vi "OPCServerSettings.vi"() -> (0 "OK Button 2":bool)   [LabVIEW 2025]
uses:
  <vilib>/Utility/config.llb/NI_LVConfig.lvlib
  <vilib>/Utility/config.llb/Write Key (String).vi
  <vilib>/Utility/config.llb/Read Key (String).vi
panel:
  in  "Cluster":cluster{"serverUrl":string, "nodeid":string}
  in  "Cancel Button":bool
  in  "OK Button":bool
  # "OPC Server settings"
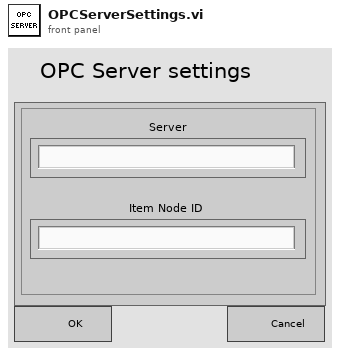
[diagram p1: front panel]
types:
  T1 = typedef "NI_LVConfig.lvlib/Config Data RefNum.ctl" = refnum<k1>
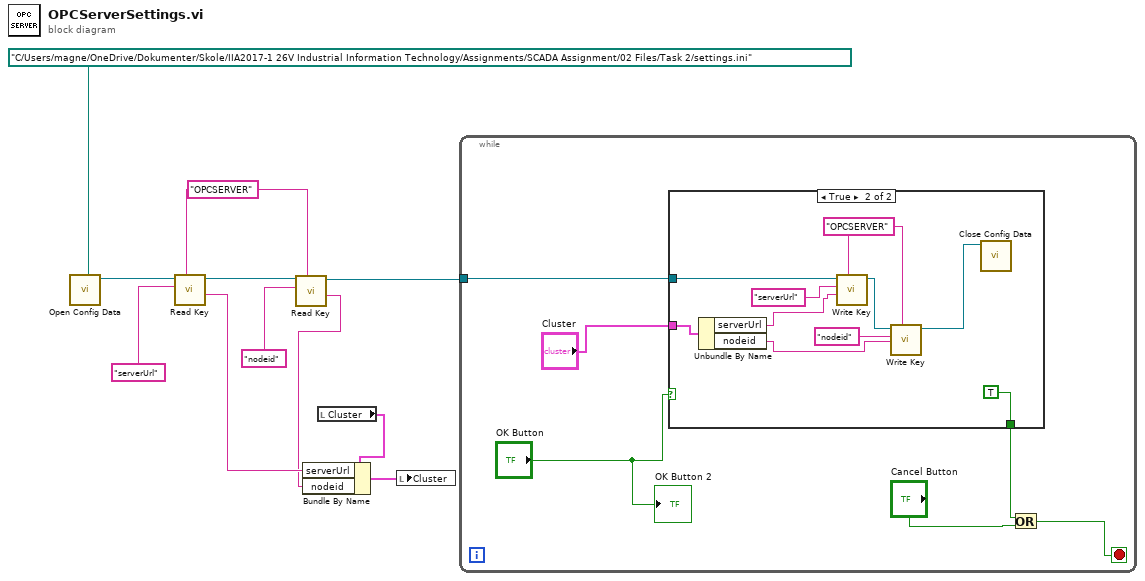
[diagram p0: block diagram]
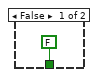
[diagram p2: hidden frame]
diagram:
  w10 = "OPCSERVER" ("section")
  n1 = call <vilib>:"Open Config Data.vi"("configuration file path"=path "C:/Users/magne/OneDrive/Dokumenter/Skole/IIA2017-1 26V Industrial Information Technology/Assignments/SCADA Assignment/02 Files/Task 2/settings.ini") -> ("refnum"=w9:T1)  [unwired: 8 in, 2 out]
  n2 = call-poly <vilib>:"Read Key.vi"("section"=w10, "key"="serverUrl", "refnum"=w9) -> ("value"=w4:string, "refnum out"=w8:T1)  [unwired: 5 in, 2 out]
  n3 = call-poly <vilib>:"Read Key.vi"("section"=w10, "key"="nodeid", "refnum"=w8) -> ("value"=w3:string, "refnum out"=w7:T1)  [unwired: 5 in, 2 out]
  n4 = local read "Cluster"() -> (w6:cluster{"serverUrl":string, "nodeid":string})
  n5 = Bundle By Name(cluster=w6, "serverUrl"=w4, "nodeid"=w3) -> (w5:cluster{"serverUrl":string, "nodeid":string})
  n6 = local write "Cluster"(w5) -> ()
  n7 = while {
    tunnel: w7 -> [w16]
    stop <- w14 stop-if-true
    n8 = case shown="True" "OK Button" {
      tunnel: "Cluster" -> [_ w28]
      tunnel: w16 -> [_ w26]
      tunnel: [FALSE ("Cancel Button") TRUE ("Cancel Button")] -> w13
      frame False {
      }
      frame True {
        w27 = "OPCSERVER" ("section")
        n9 = Unbundle By Name(w28) -> ("serverUrl"=w20:string, "nodeid"=w19:string)
        n10 = call-poly <vilib>:"Write Key.vi"("section"=w27, "value"=w20, "key"="serverUrl", "refnum"=w26) -> ("refnum out"=w25:T1)  [unwired: 5 in, 2 out]
        n11 = call-poly <vilib>:"Write Key.vi"("section"=w27, "value"=w19, "key"="nodeid", "refnum"=w25) -> ("refnum out"=w22:T1)  [unwired: 5 in, 2 out]
        n12 = call <vilib>:"Close Config Data.vi"("refnum"=w22) -> ()  [unwired: 9 in, 2 out]
      }
    }
    n13 = Or(x=w13, y="Cancel Button") -> (x .or. y?=w14:bool)
    "OK Button 2" <- "OK Button"
  }
